vi "CTemp.vi"(0 "VisaCluster":T1, 7 "CTemp":bool, 11 "error in (no error)":errorcluster) -> (4 "VisaCluster":T1, 6 "Answer":string, 8 "CTemp 2":bool, 15 "error out":errorcluster)   [LabVIEW 2014, in "FH 55.lvlib"]
doc: "This VI sets the Temp. Correction ON or OFF. \n\nDurch dieses VI kann die Temperaturkorrektur an oder abgeschaltet werden. Die Temperaturkorrektur korrigiert die Temperaturabhängigkeit der Sondenempfindlichkeit und der Offsetspannung."
uses:
  FH 55.lvlib
  TypeDef/VisaCluster.ctl
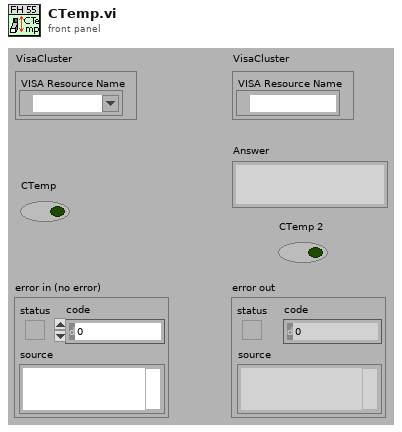
[diagram p1: front panel]
types:
  T1 = typedef "FH 55.lvlib/VisaCluster.ctl" = cluster{"VISA Resource Name":refnum<visa-resource-name>}
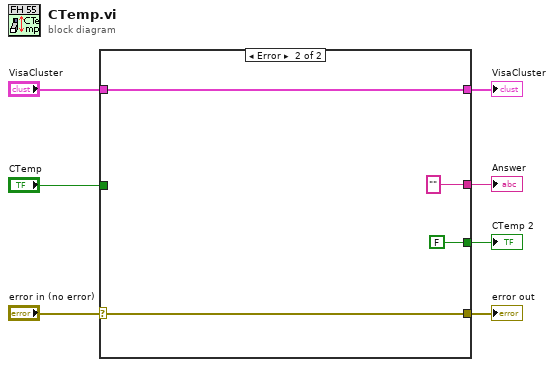
[diagram p0: block diagram]
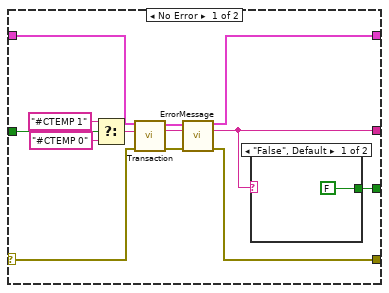
[diagram p2: hidden frame]
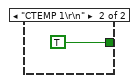
[diagram p3: hidden frame]
diagram:
  n1 = case shown="Error" "error in (no error)" {
    selector: "error in (no error)" -> [w13 w25]
    tunnel: "VisaCluster" -> [w15 w26]
    tunnel: "CTemp" -> [w20 _]
    tunnel: [w17 w26] -> w3
    tunnel: [w16 w25] -> w5
    tunnel: [w9 ""] -> w4
    tunnel: [w8 FALSE] -> w1
    frame No Error {
      n2 = Select(t="#CTEMP 1", s=w20, f="#CTEMP 0") -> (s? t:f=w14:string)
      n3 = call "Transaction.vi"("VisaCluster"=w15, "Command"=w14, "error in (no error)"=w13) -> ("VisaCluster"=w10:T1, "Answer"=w11:string, "error out"=w12:errorcluster)  [unwired: 9 in, 1 out]
      n4 = call "ErrorMessage.vi"("VisaCluster"=w10, "Message In"=w11, "error in (no error)"=w12) -> ("VisaCluster"=w17:T1, "Message Out"=w9:string, "error out"=w16:errorcluster)  [unwired: 10 in]
      n5 = case shown="\"False\", Default" w9 {
        tunnel: [FALSE TRUE] -> w8
        frame "False", Default {
        }
        frame "CTEMP 1\r\n" {
        }
      }
    }
    frame Error {
    }
  }
  "error out" <- w5
  "Answer" <- w4
  "VisaCluster" <- w3
  "CTemp 2" <- w1
